vi "Finite Sound Input.vi"() -> ()   [LabVIEW 2017]
doc: "本VI说明了从指定设备采集有限声音采样的方式。需要使用连接至声卡的麦克风。可指定需采集的采样数、采样率、通道数和每采样比特率。"
uses:
  <vilib>/sound2/lvsound2.llb/Sampling Mode.ctl
  <vilib>/sound2/lvsound2.llb/Sound Data Format.ctl
  <vilib>/sound2/lvsound2.llb/Sound Input Read (DBL).vi
panel:
  in  "设备ID":u32
  out "声音输入":waveform(dbl)[](graph)
  in  "每通道采样数":i32=10000
  # "概述：演示通过声音函数从连接至声卡的麦克风采集有限数量的的采样。\n要求：麦克风\n操作步骤：\n1.指定设备ID和每通道采样数的值。\n2.运行VI。"
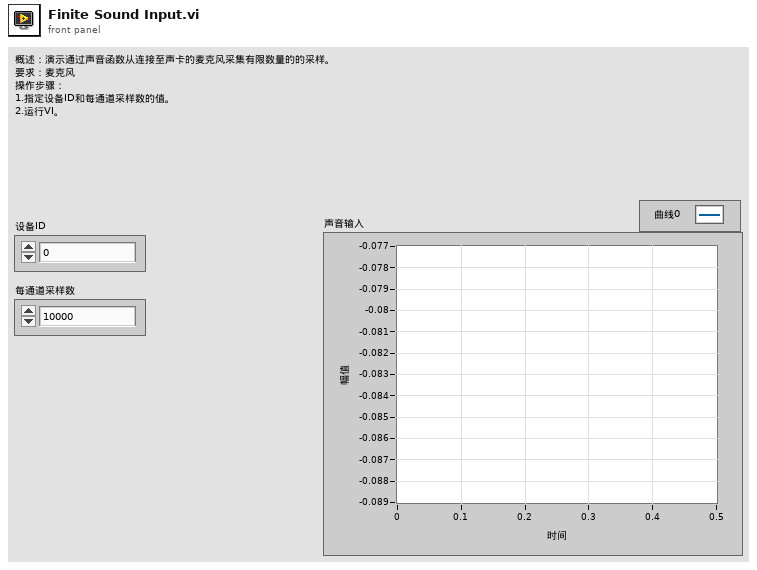
[diagram p1: front panel]
types:
  T1 = typedef "Sound Data Format.ctl" = cluster{"sample rate (S/s)":dbl, "number of channels":i32, "bits per sample":i32}
  T2 = typedef "Sampling Mode.ctl" = i32
  T3 = typedef "Sound Input Task ID.ctl" = u32
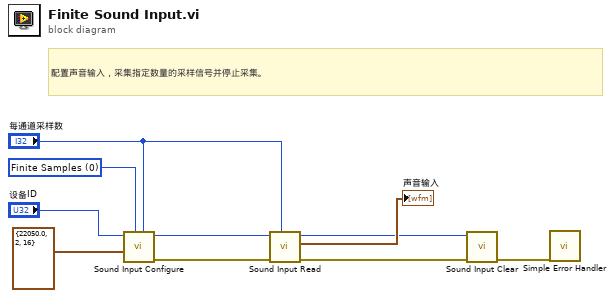
[diagram p0: block diagram]
diagram:
  w6 = T2 0 items=["Finite Samples", "Continuous Samples"] ("sample mode")
  # "配置声音输入，采集指定数量的采样信号并停止采集。"
  n1 = call <vilib>:"Sound Input Configure.vi"("number of samples/ch"="每通道采样数", "sample mode"=w6, "sound format"=T1 {"sample rate (S/s)"=22050.0, "number of channels"=2, "bits per sample"=16} ("Sound Format"), "device ID"="设备ID") -> ("error out"=w9:errorcluster, "task ID"=w7:T3)  [unwired: 6 in]
  n2 = call-poly <vilib>:"Sound Input Read.vi"("number of samples/ch"="每通道采样数", "error in (no error)"=w9, "task ID"=w7) -> ("error out"=w4:errorcluster, "data"=→"声音输入":waveform(dbl)[], "task ID out"=w5:T3)  [unwired: 6 in]
  n3 = call <vilib>:"Sound Input Clear.vi"("error in (no error)"=w4, "task ID"=w5) -> ("error out"=w1:errorcluster)  [unwired: 9 in]
  n4 = call <vilib>:"Simple Error Handler.vi"("error in (no error)"=w1) -> ()  [unwired: 4 in, 5 out]
